vi "Autosetup.vi"(8 "error in (no error)":errorcluster, 11 "TDS 2000 in":refnum<class "TDS 2000.lvclass">) -> (0 "error out":errorcluster, 3 "TDS 2000 out":refnum<class "TDS 2000.lvclass">)   [LabVIEW 2020, in "Oscilloscope.lvlib" / "TDS 2000.lvclass"]
uses:
  TDS 2000.lvclass
  C:/Users/ronad/Osciloscopio/Osciloscopio DQMH/Libraries/Oscilloscope/Clases/Osciloscopio/Osciloscopio.lvclass
  Osciloscopio/Osciloscopio.lvclass/Osciloscopio.ctl
  Osciloscopio/Read COM.vi
  Osciloscopio/Write COM.vi
  <instrlib>/Tektronix TDS 200 1000 2000 Series/Tektronix TDS 200 1000 2000 Series.lvlib
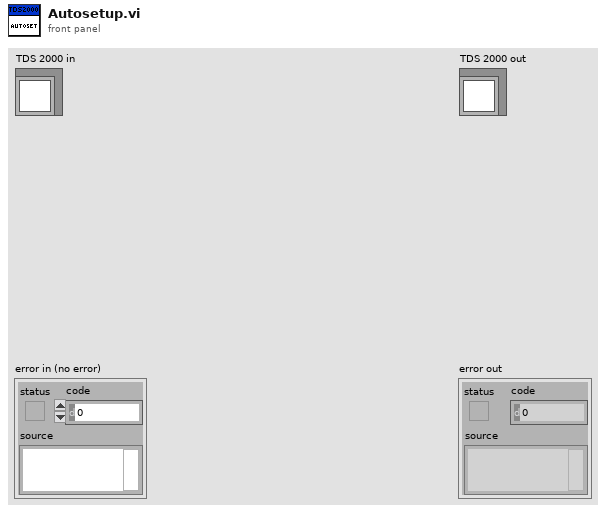
[diagram p1: front panel]
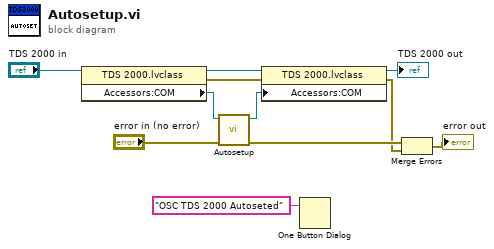
[diagram p0: block diagram]
diagram:
  n1 = property class="TDS 2000.lvclass"(reference="TDS 2000 in") -> (reference out=w8:refnum<class "TDS 2000.lvclass">, error out=w4:errorcluster, "Accessors:COM"=w10:refnum<visa-resource-name>)  [unwired: 1 in]
  n2 = call <instrlib>:"Autosetup.vi"("error in (no error)"="error in (no error)", "VISA resource name"=w10) -> ("error out"=w6:errorcluster, "VISA resource name out"=w9:refnum<visa-resource-name>)  [unwired: 8 in]
  n3 = property class="TDS 2000.lvclass"(reference=w8, error in=w4, "Accessors:COM"=w9) -> (reference out=→"TDS 2000 out":refnum<class "TDS 2000.lvclass">, error out=w2:errorcluster)
  n4 = One Button Dialog(message="OSC TDS 2000 Autoseted") -> ()  [unwired: 1 in, 1 out]
  n5 = Merge Errors(w6, w2) -> (→"error out":errorcluster)
